vi "SystemDataPanel.vi"() -> ()   [LabVIEW 2019]
uses:
  <vilib>/Utility/miscctls.llb/LVPositionTypeDef.ctl
  Ctrl/System Data Action.ctl
  <vilib>/Utility/miscctls.llb/LVPointTypeDef.ctl
  LLB/Message/Ctrl/MsgDataInput.ctl
  LLB/Message/Ctrl/MsgPageSelect.ctl
  LLB/Message/Ctrl/LogType.ctl
  LLB/Message/MsgShowAndLog.lvlib
  LLB/Commonly VI.lvlib
panel:
  in  "$VISA resource name":refnum<visa-resource-name>
  in  "$Ring":u16(ring) caption="Ring" items=["A", "V", "C"]
  in  "$VType":enum16{"無條件捨去", "四捨五入"}(ring) caption="電壓選取方式"
  in  "$ForceSetBinChk_":bool caption="使用手動參數"
  in  "$Bin V DiffNum_":dbl caption="電壓差(V)" min=0.0 step=0.001 format="%#_4g"
  in  "$Standar VNum_":string caption="標準電壓"
  in  "Variant":variant
  in  "Tab Control":refnum<vi>
  out "Class ID":u32
  out "Class Name":string
  out "OldVal":variant
  out "NewVal":variant
  in  "SData_VisionRef":T1 caption="VisionRef"
  in  "Tab Control 2":enum32{"Page 1"}(tab)
  in  "Save":bool
  # "自動計算規則"
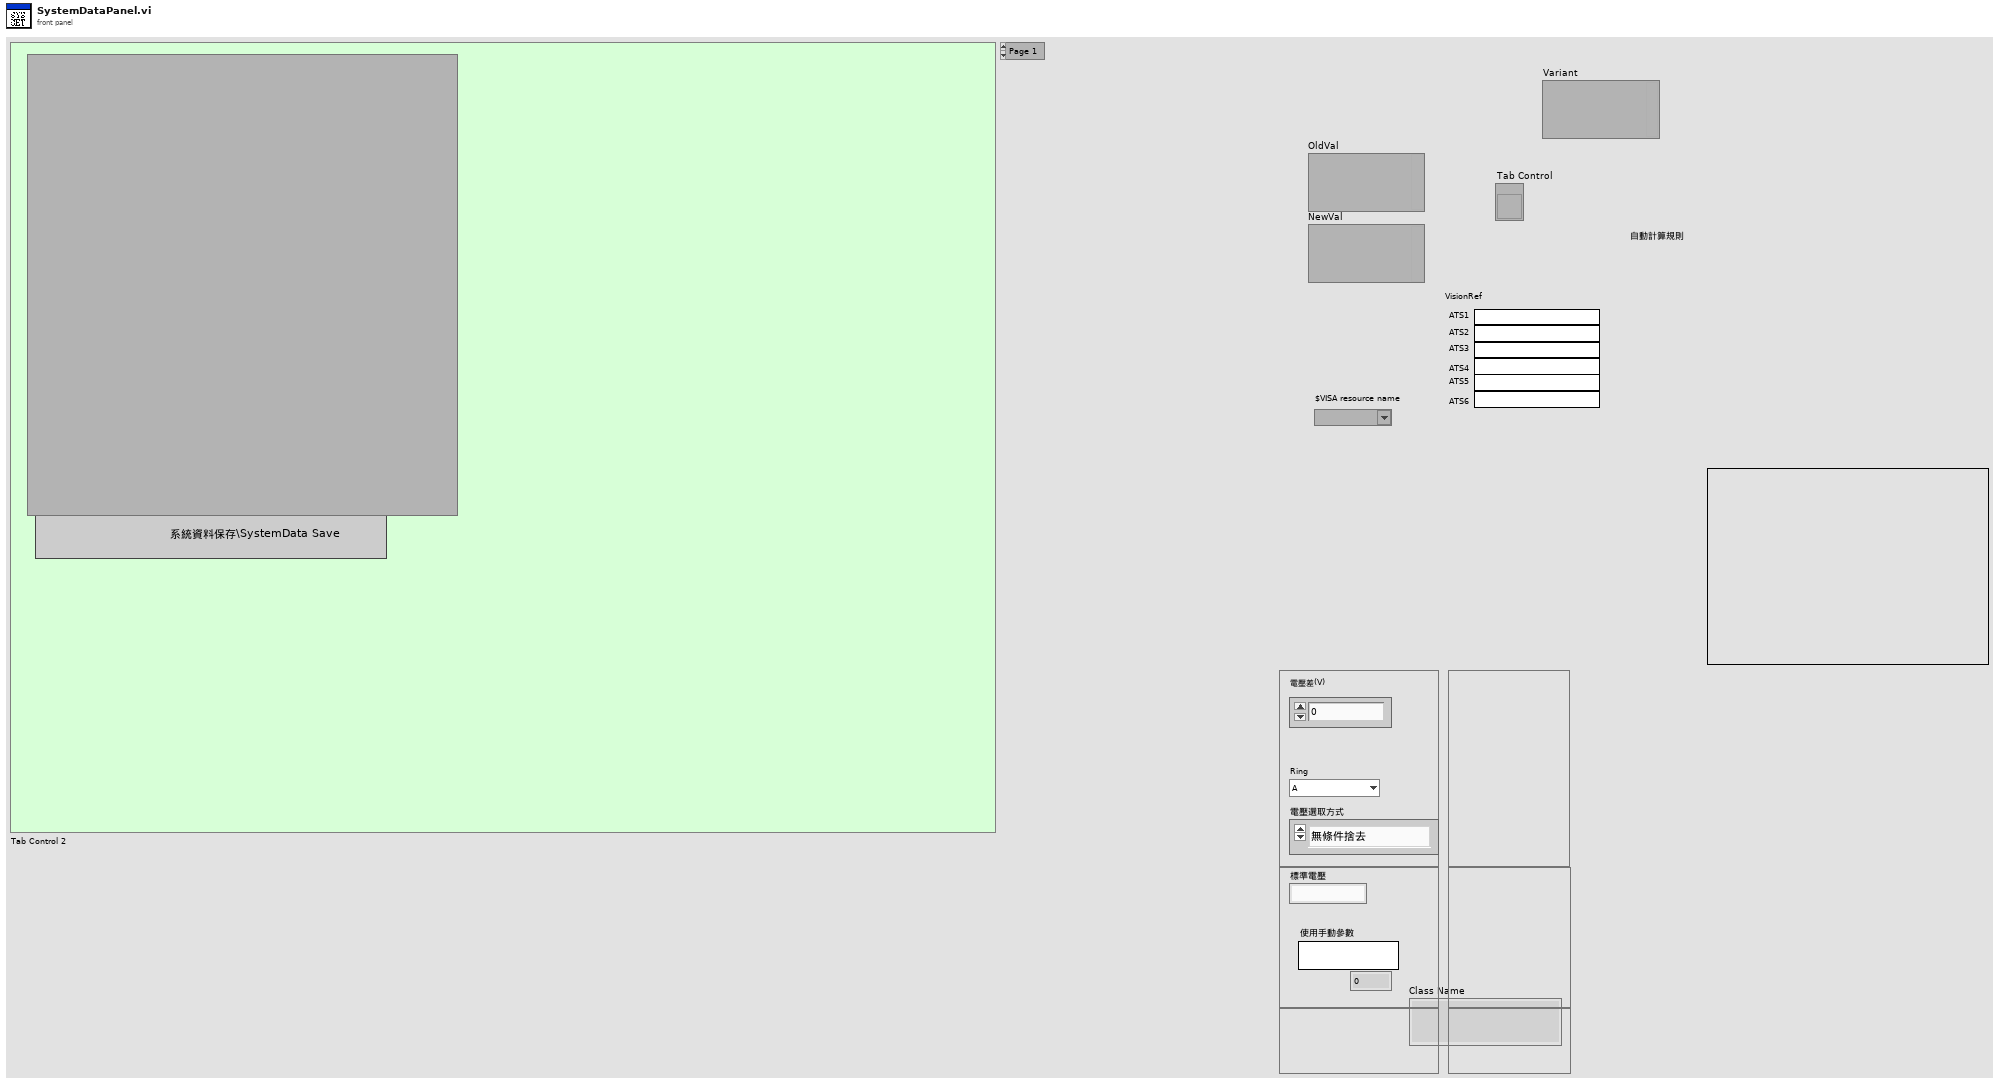
[diagram p1: front panel]
types:
  T1 = cluster{"ATS1":string, "ATS2":string, "ATS3":string, "ATS4":string, "ATS5":string, "ATS6":string, "SHB7":string, "SHB8":string}
  T2 = typedef "LVPositionTypeDef.ctl" = cluster{"Left":i32, "Top":i32}
  T3 = typedef "System Data Action.ctl" = enum16{"initial", "save", "load", "write", "read"}
  T4 = typedef "LVPointTypeDef.ctl" = cluster{"Horizontal":i16, "Vertical":i16}
  T5 = typedef "MsgDataInput.ctl" = cluster{"MsgPageSelect":T6, "LogType":T7, "Msg":string, "Time":string}
  T6 = typedef "MsgShowAndLog.lvlib/MsgPageSelect.ctl" = enum16{"System", "Comm", "IO", "Action", "Alarm"}
  T7 = typedef "MsgShowAndLog.lvlib/LogType.ctl" = enum16{"Auto", "Manual", "Handshake", "Error"}
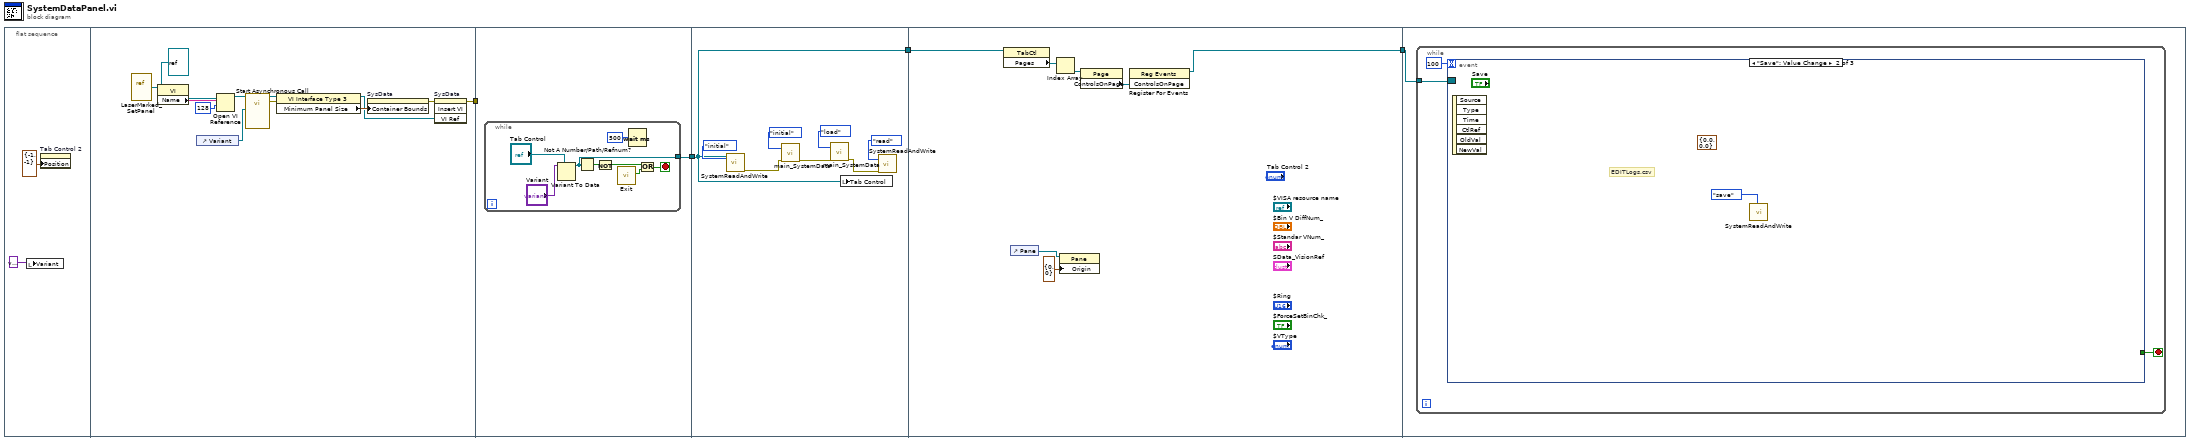
[diagram p0: block diagram]
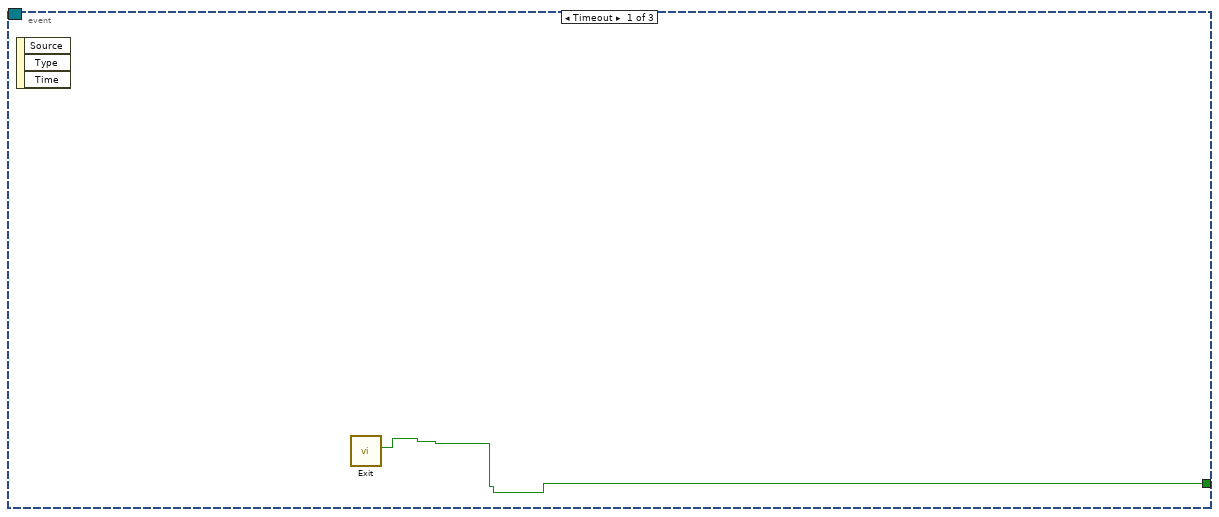
[diagram p2: hidden frame]
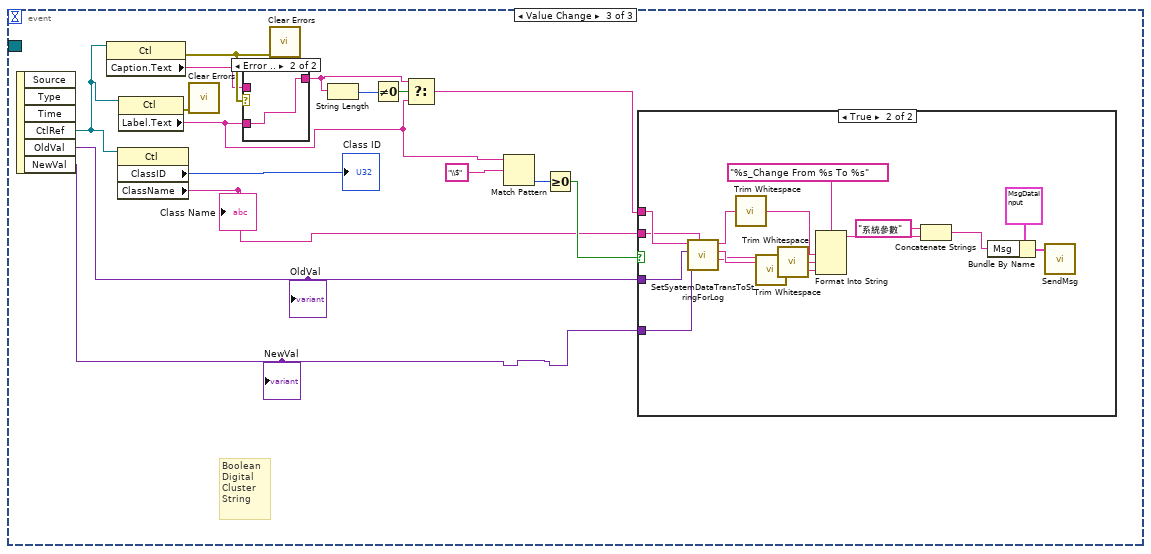
[diagram p3: hidden frame]
diagram:
  n1 = flat-sequence {
    tunnel: [w8] -> w1
    tunnel: [w19] -> w3
    tunnel: w1 -> [_]
    tunnel: w3 -> [w33]
    tunnel: [w33] -> w2
    tunnel: [w42] -> w4
    tunnel: w2 -> [w38]
    tunnel: w4 -> [w43]
    frame #0 {
      n2 = local write "Variant"(variant) -> ()
      n3 = property on="Tab Control 2" class="TabCtl (strict)"("Position"=T2 {"Left"=-1, "Top"=-1}) -> ()  [unwired: 2 in, 2 out]
    }
    frame #1 {
      n4 = vi-ref "LaserMarked_SetPanel.vi"() -> (w7:refnum<vi>)
      n5 = property class="VI"(reference=w7) -> ("Name"=w18:string)  [unwired: 1 in, 2 out]
      n6 = control-ref of="Variant"() -> (w9:refnum<vi>)
      n7 = Open VI Reference(type specifier VI Refnum (for type only)=refnum<vi> refnum, vi path=w18, options=128) -> (vi reference=w16:refnum<vi>)  [unwired: 3 in, 1 out]
      n8 = call-by-ref "Start Asynchronous Call"(reference=w16, "SetPanelRef"=w9) -> (reference out=w15:refnum<vi>, error out=w14:errorcluster)  [unwired: 12 in]
      n9 = property class="VI Interface Type 3"(reference=w15, error in=w14) -> (reference out=w12:refnum<vi>, "Minimum Panel Size"=w13:T4)  [unwired: 1 out]
      n10 = property on="SysData" class="SubPnl"("Container Bounds"=w13) -> (error out=w11:errorcluster)  [unwired: 2 in, 1 out]
      n11 = invoke on="SysData" class="SubPnl" method="Insert VI"(error in=w11, "VI Ref"=w12) -> (error out=w8:errorcluster)  [unwired: 2 in, 3 out]
    }
    frame #2 {
      n12 = while {
        tunnel: [w25] -> w19
        stop <- w23 stop-if-true
        n13 = Variant To Data(type="Tab Control", Variant="Variant") -> (data=w25:refnum<vi>)  [unwired: 1 in, 1 out]
        n14 = Not A Number/Path/Refnum?(number/path/refnum=w25) -> (NaN/Path/Refnum?=w24:bool)
        n15 = Not(x=w24) -> (.not. x?=w21:bool)
        n16 = call "Exit.vi"() -> ("ExitOut"=w22:bool)  [unwired: 11 in]
        n17 = Wait (ms)(milliseconds to wait=u32 500) -> ()  [unwired: 1 out]
        n18 = Or(x=w21, y=w22) -> (x .or. y?=w23:bool)
      }
    }
    frame #3 {
      n19 = call "SystemReadAndWrite.vi"("Enum"=enum16{"initial", "save", "read"}."initial", "Tab Control"=w33) -> ("error out"=w29:errorcluster)  [unwired: 9 in]
      n20 = call "main_SystemData.vi"("Enum"=System_Data_Action."initial", "error in"=w29) -> ("error out"=w30:errorcluster)  [unwired: 7 in, 2 out]
      n21 = call "main_SystemData.vi"("Enum"=System_Data_Action."load", "error in"=w30) -> ("error out"=w28:errorcluster)  [unwired: 7 in, 2 out]
      n22 = local write "Tab Control"(w33) -> ()
      n23 = call "SystemReadAndWrite.vi"("Enum"=enum16{"initial", "save", "read"}."read", "error in"=w28) -> ()  [unwired: 9 in, 1 out]
    }
    frame #4 {
      n24 = property class="TabCtl"(reference=w38) -> ("Pages"=w41:refnum<vi>[])  [unwired: 1 in, 2 out]
      n25 = control-ref of="Pane"() -> (w37:refnum<vi>)
      n26 = Index Array(array=w41) -> (element=w40:refnum<vi>)  [unwired: 1 in]
      n27 = property class="Pane"(reference=w37, "Origin"=T4 {"Horizontal"=0, "Vertical"=0}) -> ()  [unwired: 1 in, 2 out]
      n28 = property class="Page"(reference=w40) -> ("ControlsOnPage"=w39:refnum<vi>[])  [unwired: 1 in, 2 out]
      n29 = register-events(w39) -> (reference out=w42:refnum<event-registration>)  [unwired: 2 in, 1 out]
    }
    frame #5 {
      n30 = while {
        tunnel: w43 -> [w44]
        stop <- w45 stop-if-true
        n31 = event shown="[1] \"Save\": Value Change" {
          selector: w44 -> [_ _ _]
          dyn-events: _ -> [_ _ _]
          timeout: 100 -> [_ _ _]
          tunnel: [w47 _ _] -> w45
          event Timeout {
            n32 = event-data() -> ()  [unwired: 1 in, 3 out]
            n33 = call "Exit.vi"() -> ("ExitOut"=w47:bool)  [unwired: 11 in]
          }
          event "Save": Value Change {
            (unwired) cluster{"Max":dbl, "Min":dbl} {"Max"=0.0, "Min"=0.0} ("BinRange")
            # "EDITLogs.csv"
            n34 = event-data() -> ()  [unwired: 1 in, 6 out]
            n35 = call "SystemReadAndWrite.vi"("Enum"=enum16{"initial", "save", "read"}."save") -> ()  [unwired: 10 in, 1 out]
          }
          event Value Change {
            # "Boolean\nDigital\nCluster\nString"
            n36 = event-data() -> ("CtlRef"=w54:refnum<vi>, "OldVal"=w59:variant, "NewVal"=w60:variant)  [unwired: 1 in, 3 out]
            "OldVal" <- w59
            "NewVal" <- w60
            n37 = property class="Ctl"(reference=w54) -> (error out=w52:errorcluster, "Caption.Text"=w50:string)  [unwired: 1 in, 1 out]
            n38 = property class="Ctl"(reference=w54) -> ("ClassID"=→"Class ID":u32, "ClassName"=w58:string)  [unwired: 1 in, 2 out]
            "Class Name" <- w58
            n39 = property class="Ctl"(reference=w54) -> (error out=w53:errorcluster, "Label.Text"=w49:string)  [unwired: 1 in, 1 out]
            n40 = call <vilib>:"Clear Errors.vi"("error in (no error)"=w53) -> ()  [unwired: 5 in, 2 out]
            n41 = case shown="Error .." w52 {
              tunnel: [w65 w66] -> w51
              tunnel: w50 -> [w65 _]
              tunnel: w49 -> [_ w66]
              frame No Error {
              }
              frame Error {
              }
            }
            n42 = call <vilib>:"Clear Errors.vi"("error in (no error)"=w52) -> ()  [unwired: 5 in, 2 out]
            n43 = String Length(string=w51) -> (length=w57:i32)
            n44 = Not Equal To 0?(x=w57) -> (x != 0?=w56:bool)
            n45 = Select(t=w51, s=w56, f=w49) -> (s? t:f=w55:string)
            n46 = Match Pattern(string=w49, regular expression="\\$") -> (offset past match=w62:i32)  [unwired: 1 in, 3 out]
            n47 = Greater Or Equal To 0?(x=w62) -> (x >= 0?=w61:bool)
            n48 = case shown="True" w61 {
              tunnel: w59 -> [_ w79]
              tunnel: w60 -> [_ w78]
              tunnel: w55 -> [_ w70]
              tunnel: w58 -> [_ w69]
              frame False {
              }
              frame True {
                n49 = call "SetSyatemDataTransToStringForLog.vi"("Class Name"=w69, "NewVal"=w78, "OldVal"=w79, "Label.Text"=w70) -> ("NewData"=w76:string, "OldData"=w77:string, "DataName"=w80:string)  [unwired: 5 in]
                n50 = call <vilib>:"Trim Whitespace.vi"("string"=w80) -> ("trimmed string"=w81:string)  [unwired: 1 in]
                n51 = call <vilib>:"Trim Whitespace.vi"("string"=w76) -> ("trimmed string"=w74:string)  [unwired: 1 in]
                n52 = call <vilib>:"Trim Whitespace.vi"("string"=w77) -> ("trimmed string"=w75:string)  [unwired: 1 in]
                n53 = Format Into String(format string="%s_Change From %s To %s", w81, w75, w74) -> (resulting string=w71:string)  [unwired: 2 in, 1 out]
                n54 = Concatenate Strings("系統參數" ("string"), w71) -> (w68:string)
                n55 = Bundle By Name(cluster=T5 {"MsgPageSelect"=enum."System", "LogType"=enum."Manual", "Msg"="刪除專案 KKI", "Time"=""} ("DataIn"), "Msg"=w68) -> (w72:T5)
                n56 = call "SendMsg.vi"("DataIn"=w72) -> ()  [unwired: 10 in, 1 out]
              }
            }
          }
        }
      }
    }
  }
